vi "Shooter Template_wrapper.vi"() -> ()   [LabVIEW 2020]
uses:
  <vilib>/Rock Robotics/WPI/Framework/Command Status Info.ctl
  <vilib>/Rock Robotics/WPI/Framework/Completion Status.ctl
  <vilib>/Rock Robotics/WPI/Framework/Completion Notifier.ctl
panel:
  in  "Description":string
  in  "hood (pos)":dbl
  in  "top flywheel (vol)":dbl
  in  "flywheel (vol)":dbl
  out "Command Info Out":T1
  in  "Command Info In":T1
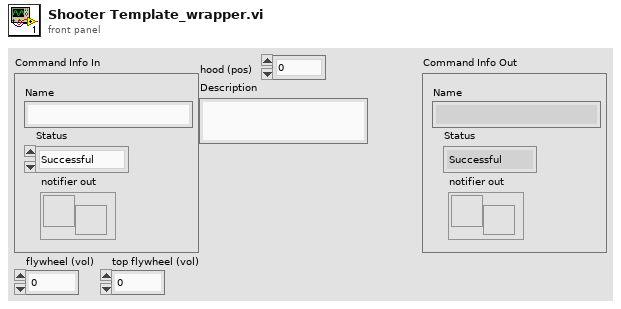
[diagram p1: front panel]
types:
  T1 = typedef "Command Status Info.ctl" = cluster{"Name":string, "Status":T2, "notifier out":T3}
  T2 = typedef "Completion Status.ctl" = enum16{"Successful", "Aborted", "Incomplete"}
  T3 = typedef "Completion Notifier.ctl" = refnum<notifier>
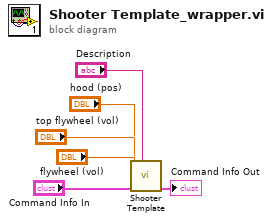
[diagram p0: block diagram]
diagram:
  n1 = call "Shooter Template.vi"("Description"="Description", "Command Info In"="Command Info In", "top flywheel (vol)"="top flywheel (vol)", "flywheel (vol)"="flywheel (vol)", "hood (pos)"="hood (pos)") -> ("Command Info Out"=→"Command Info Out":T1)  [unwired: 6 in]
